vi "Send Message and Wait for Response.vi"(6 "DataSocket Location":string="dstp://localhost/fan1", 7 "Message Priority (Normal)":T1=enum."Normal", 8 "error in":errorcluster, 9 "timeout in ms (-1)":i32=-1, 10 "Original Message":refnum<class "DS Reply Msg.lvclass">, 11 "Message Enqueuer in":refnum<class "Message Enqueuer.lvclass">) -> (0 "error out":errorcluster, 1 "timed out?":bool, 2 "Reply":variant, 3 "Message Enqueuer out":refnum<class "Message Enqueuer.lvclass">)   [LabVIEW 2023, in "DS Reply Msg.lvclass"]
uses:
  DS Reply Msg.lvclass
  <vilib>/ActorFramework/Message Enqueuer/Message Enqueuer.lvclass
  <vilib>/ActorFramework/Message Enqueuer/Message Priority.ctl
  C:/Program Files/National Instruments/LabVIEW 2023/vi.lib/ActorFramework/Message/Message.lvclass
  DS Reply Msg.lvclass/DS Reply Msg.ctl
  <vilib>/ActorFramework/Message Enqueuer/Message Enqueuer.lvclass/Message Enqueuer.ctl
  <vilib>/Utility/LVClass/Get LV Class Name.vi
  <resource>/AFDebug/Generate Trace for Message.vi
  <vilib>/ActorFramework/Message Priority Queue/Priority Enqueue.vi
  D:/git/DS-Reply-Msg/DS Reply Msg/DS Reply Msg.lvclass
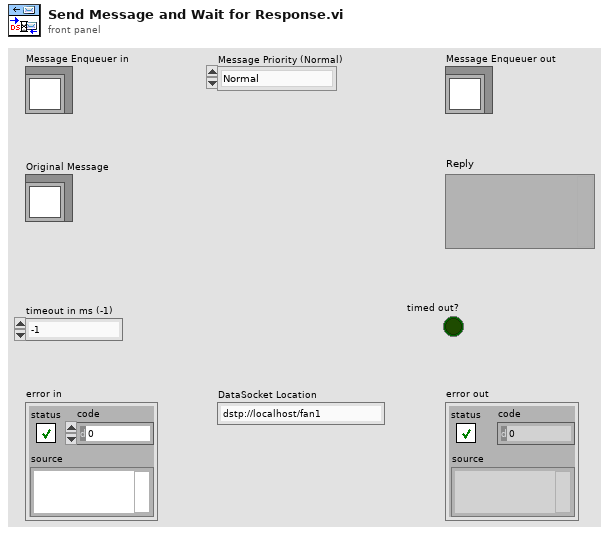
[diagram p1: front panel]
types:
  T1 = typedef "Actor Framework.lvlib/Message Enqueuer.lvclass/Message Priority.ctl" = enum16{"Low", "Normal", "High"}
  T2 = enum16{"Read", "Write", "ReadWrite", "BufferedRead", "BufferedReadWrite"}
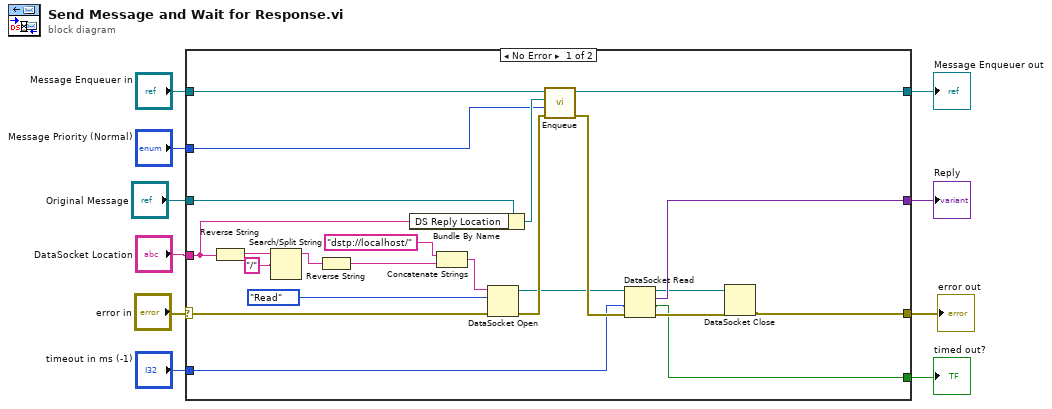
[diagram p0: block diagram]
diagram:
  n1 = case shown="No Error" "error in" {
    selector: "error in" -> [w28 w35]
    tunnel: [w21 w35] -> w3
    tunnel: "Original Message" -> [w18 _]
    tunnel: "Message Enqueuer in" -> [w33 w34]
    tunnel: [w23 _] -> w6
    tunnel: "timeout in ms (-1)" -> [w25 _]
    tunnel: [w20 _] -> w9
    tunnel: "Message Priority (Normal)" -> [w31 _]
    tunnel: [w30 w34] -> w5
    tunnel: "DataSocket Location" -> [w15 _]
    frame No Error {
      n2 = Reverse String(1:w15) -> (0:w14:string)
      n3 = Search/Split String(string=w14, search string/char (-)="/") -> (substring before match=w12:string)  [unwired: 1 in, 2 out]
      n4 = Reverse String(1:w12) -> (0:w11:string)
      n5 = Bundle By Name(cluster=w18, "DS Reply Location"=w15) -> (w32:refnum<class "DS Reply Msg.lvclass">)
      n6 = Concatenate Strings("dstp://localhost/", w11) -> (w16:string)
      n7 = DataSocket Open(8:w28, 10:T2."Read" ("mode"), 11:w16) -> (0:w27:errorcluster, 3:w24:refnum<k13>)  [unwired: 1 in]
      n8 = call <vilib>:"Enqueue.vi"("error in (no error)"=w27, "Message Priority (Normal)"=w31, "Message"=w32, "Message Enqueuer in"=w33) -> ("error out"=w26:errorcluster, "Message Enqueuer out"=w30:refnum<class "Message Enqueuer.lvclass">)  [unwired: 6 in]
      n9 = DataSocket Read(8:w26, 9:w25, 11:w24) -> (0:w22:errorcluster, 1:w20:bool, 2:w23:variant, 3:w19:refnum<k13>)  [unwired: 1 in, 4 out]
      n10 = DataSocket Close(8:w22, 11:w19) -> (0:w21:errorcluster)  [unwired: 1 in, 1 out]
    }
    frame Error {
    }
  }
  "error out" <- w3
  "timed out?" <- w9
  "Reply" <- w6
  "Message Enqueuer out" <- w5
